vi "SortAlphabetically.vi"(8 "error in":errorcluster, 9 "TreeSectHdrs":string, 11 "FrameNames":string[](array[string])) -> (0 "error out":errorcluster, 3 "Sorted":i32[](array[numeric]))   [LabVIEW 2020]
doc: "This VI will sort an array of FrameNames alphabetically, first by section headers then within each header. If no headers are defined it will simply sort them alphabetically. It returns an array of indices of the items in FrameNames as they will be after being sorted. It will leave the first case first if it's not in a section (ex. Idle case in a JKI State Machine)."
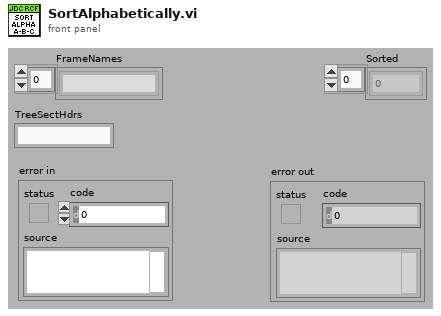
[diagram p1: front panel]
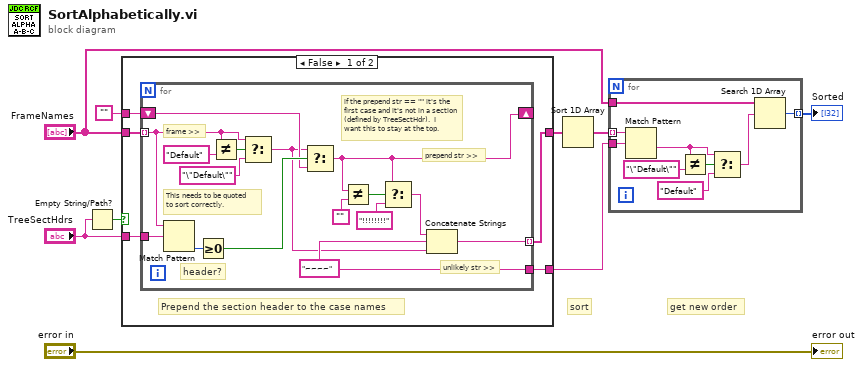
[diagram p0: block diagram]
diagram:
  # "get new order"
  # "sort"
  n1 = Empty String/Path?(string/path="TreeSectHdrs") -> (empty?=w9:bool)
  n2 = case shown="False" w9 {
    tunnel: [w11 w31] -> w6
    tunnel: "FrameNames" -> [w14 w31]
    tunnel: "TreeSectHdrs" -> [w13 _]
    tunnel: "" -> [w12 _]
    tunnel: [w10 _] -> w7
    frame False {
      # "Prepend the section header to the case names"
      n3 = for {
        tunnel: w14 -> [w21] mode=indexing
        tunnel: w13 -> [w30]
        shift-right: [w17] -> _
        shift-left: w12 -> [w27]
        tunnel: [w26] -> w11 mode=indexing
        tunnel: [w25] -> w10
        w25 = "~~~~" ("string")
        # "if the prepend str == \"\" it's the\nfirst case and it's not in a section\n(defined by TreeSectHdr).  I \nwant this to stay at the top."
        # "This needs to be quoted\nto sort correctly."
        # "unlikely str >>"
        # "frame >>"
        # "prepend str >>"
        # "header?"
        n4 = Match Pattern(string=w21, regular expression=w30) -> (offset past match=w29:i32)  [unwired: 4 out]
        n5 = Greater Or Equal To 0?(x=w29) -> (x >= 0?=w28:bool)
        n6 = Not Equal?(x=w21, y="Default") -> (x != y?=w23:bool)
        n7 = Select(t=w21, s=w23, f="\"Default\"") -> (s? t:f=w20:string)
        n8 = Select(t=w20, s=w28, f=w27) -> (s? t:f=w17:string)
        n9 = Not Equal?(x=w17, y="") -> (x != y?=w18:bool)
        n10 = Select(t=w17, s=w18, f="!!!!!!!!") -> (s? t:f=w16:string)
        n11 = Concatenate Strings(w16, w25, w20) -> (w26:string)
      }
    }
    frame True {
      # "Nothing to do here...  Move along!"
    }
  }
  n12 = Sort 1D Array(array=w6) -> (sorted array=w5:string[])
  n13 = for {
    tunnel: w5 -> [w39] mode=indexing
    tunnel: "FrameNames" -> [w40]
    tunnel: w7 -> [w38]
    tunnel: [w37] -> w2 mode=indexing
    n14 = Match Pattern(string=w39, regular expression=w38) -> (after substring=w33:string)  [unwired: 4 out]
    n15 = Not Equal?(x=w33, y="\"Default\"") -> (x != y?=w35:bool)
    n16 = Select(t=w33, s=w35, f="Default") -> (s? t:f=w32:string)
    n17 = Search 1D Array(1D array=w40, element=w32) -> (index of element=w37:i32)  [unwired: 1 out]
  }
  "Sorted" <- w2
  "error out" <- "error in"
